vi "TemperatureEng.vi"(5 "Set Temperature":dbl, 6 "Action":enum16{"Set Celsius", "Get Temps"}(ring)) -> (0 "Output3":sgl, 1 "Output2":sgl, 2 "Output1":sgl, 3 "Error":bool, 4 "Output4":sgl)   [LabVIEW 2014]
panel:
  # "C"
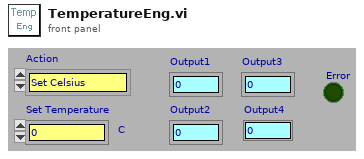
[diagram p1: front panel]
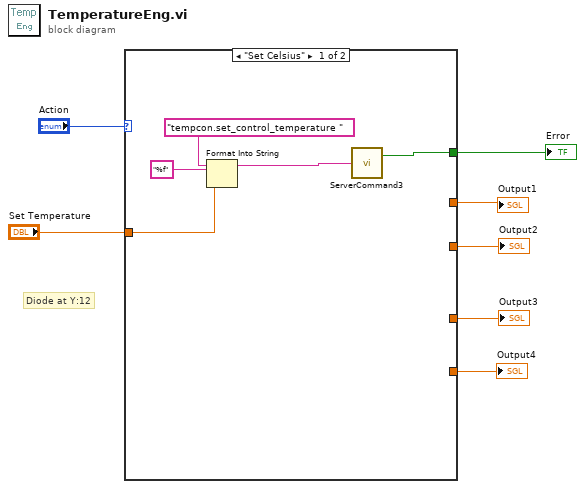
[diagram p0: block diagram]
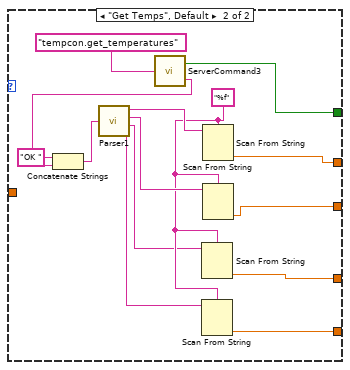
[diagram p2: hidden frame]
diagram:
  # "Diode at Y:12"
  n1 = case shown="\"Set Celsius\"" "Action" {
    tunnel: [_ w25] -> w6
    tunnel: "Set Temperature" -> [w12 _]
    tunnel: [_ w26] -> w4
    tunnel: [w9 w18] -> w3
    tunnel: [_ w14] -> w2
    tunnel: [_ w13] -> w1
    frame "Set Celsius" {
      n2 = Format Into String(format string="%f", initial string="tempcon.set_control_temperature " ("Command"), w12) -> (resulting string=w8:string)  [unwired: 1 in, 1 out]
      n3 = call "ServerCommand3.vi"("Command"=w8) -> ("Error"=w9:bool)  [unwired: 1 out]
    }
    frame "Get Temps", Default {
      w17 = "%f" ("format string")
      n4 = call "ServerCommand3.vi"("Command"="tempcon.get_temperatures") -> ("Error"=w18:bool, "Reply"=w20:string)
      n5 = Concatenate Strings("OK " ("string"), w20) -> (w19:string)
      n6 = call "Parser1.vi"("InputString"=w19) -> ("Arg1 Out"=w23:string, "Arg2 Out"=w22:string, "Arg3 Out"=w16:string, "Arg4 Out"=w15:string)  [unwired: 2 out]
      n7 = Scan From String(format string=w17, input string=w16) -> (output 1=w14:dbl)  [unwired: 3 in, 3 out]
      n8 = Scan From String(format string=w17, input string=w15) -> (output 1=w13:dbl)  [unwired: 3 in, 3 out]
      n9 = Scan From String(format string=w17, input string=w23) -> (output 1=w25:dbl)  [unwired: 3 in, 3 out]
      n10 = Scan From String(format string=w17, input string=w22) -> (output 1=w26:dbl)  [unwired: 3 in, 3 out]
    }
  }
  "Output1" <- w6
  "Output2" <- w4
  "Error" <- w3
  "Output3" <- w2
  "Output4" <- w1
